vi "Send_Command.vi"(7 "port":u16=6379, 8 "error in":errorcluster, 10 "command":string="PING", 11 "host":string="localhost") -> (0 "error out":errorcluster, 1 "string data":string[](array[string]), 2 "reply":T1, 3 "type":T2(ring))   [LabVIEW 2023]
uses:
  SubVIs/Controls/redis-type.ctl
panel:
  out "string":string
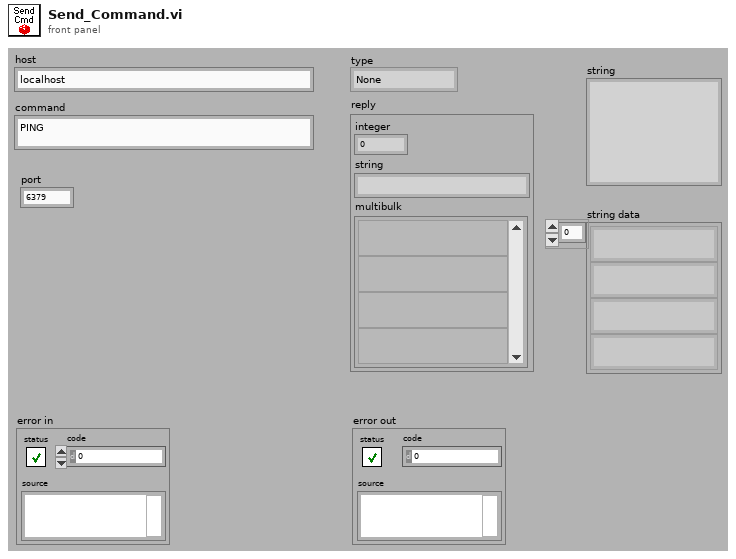
[diagram p1: front panel]
types:
  T1 = cluster{"integer":i64, "string":string, "multibulk":variant[]}
  T2 = enum16{"None", "Error", "Status", "Nil", "Integer", "String", "Multibulk"}
  T3 = typedef "redis-type.ctl" = enum16{"None", "Error", "Status", "Nil", "Integer", "String", "Multibulk"}
  T4 = typedef "redis-reply.ctl" = cluster{"integer":i64, "string":string, "multibulk":variant[]}
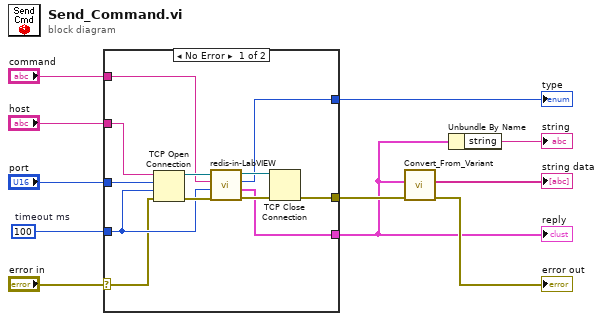
[diagram p0: block diagram]
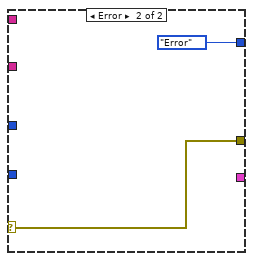
[diagram p2: hidden frame]
diagram:
  w9 = 100  # timeout ms
  n1 = case shown="No Error" "error in" {
    selector: "error in" -> [w14 w24]
    tunnel: "port" -> [w23 _]
    tunnel: [w21 redis-type."Error" ("reply type")] -> w11
    tunnel: [w13 _] -> w2
    tunnel: "host" -> [w20 _]
    tunnel: w9 -> [w16 _]
    tunnel: "command" -> [w15 _]
    tunnel: [w12 w24] -> w4
    frame No Error {
      n2 = TCP Open Connection(address=w20, remote port or service name=w23, timeout ms (60000)=w16, error in (no error)=w14) -> (connection ID=w18:refnum<k5>, error out=w17:errorcluster)  [unwired: 1 in]
      n3 = call "redis-in-LabVIEW.vi"("Error in"=w17, "Timeout ms"=w16, "Command"=w15, "TCP in"=w18) -> ("Error out"=w19:errorcluster, "redis reply"=w13:T4, "reply type"=w21:T3, "TCP out"=w22:refnum<k5>)
      n4 = TCP Close Connection(connection ID=w22, error in (no error)=w19) -> (error out=w12:errorcluster)  [unwired: 1 in, 1 out]
    }
    frame Error {
    }
  }
  "type" <- w11
  "reply" <- w2
  n5 = call "Convert_From_Variant.vi"("error in"=w4, "Data in"=w2) -> ("error out"=→"error out":errorcluster, "String data out"=→"string data":string[])  [unwired: 8 in]
  n6 = Unbundle By Name(w2) -> ("string"=→"string":string)
